vi "Leak Actor State.vi"(8 "error in (no error)":errorcluster, 11 "ViewableOne in":refnum<class "LeakyViewable.lvclass">) -> (0 "error out":errorcluster, 3 "ViewableOne out":refnum<class "LeakyViewable.lvclass">)   [LabVIEW 2017, in "ViewableDoubles.lvlib" / "LeakyViewable.lvclass"]
uses:
  LeakyViewable.lvclass
  C:/Git/mva-framework/Framework/IViewable/IViewable/IViewable.lvclass
  LeakyViewable.lvclass/LeakyViewable.ctl
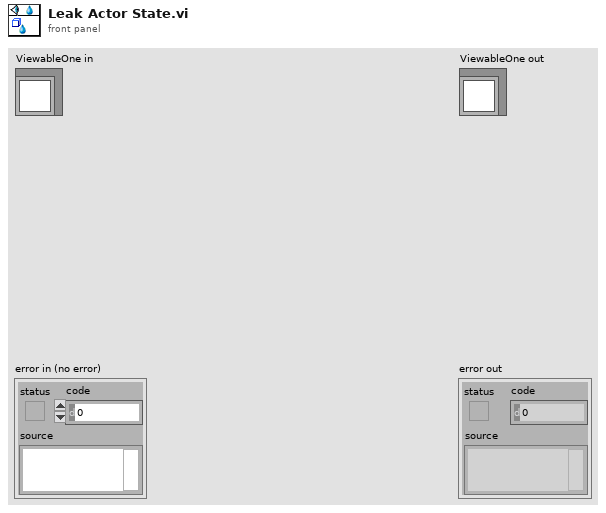
[diagram p1: front panel]
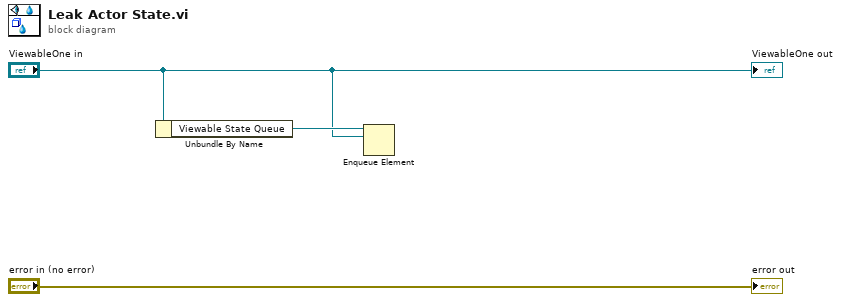
[diagram p0: block diagram]
diagram:
  n1 = Unbundle By Name("ViewableOne in") -> ("Viewable State Queue"=w2:refnum<queue>)
  n2 = Enqueue Element(queue=w2, element="ViewableOne in") -> ()  [unwired: 2 in, 3 out]
  "error out" <- "error in (no error)"
  "ViewableOne out" <- "ViewableOne in"
